vi "2D array to IMAQ.vi"(7 "Image Pixels (U8)":u8[][](array[numeric]), 8 "error in (no error)":errorcluster, 9 "Image Name":string="untitled", 10 "Image":T1, 11 "Thorcam in":refnum<class "Thorcam.lvclass">) -> (0 "error out":errorcluster, 2 "Image Name 2":string, 3 "Thorcam out":refnum<class "Thorcam.lvclass">, 4 "Image Out":T1)   [LabVIEW 2012, in "Thorcam.lvclass"]
uses:
  Thorcam.lvclass
  <vilib>/vision/Image Controls.llb/IMAQ Image.ctl
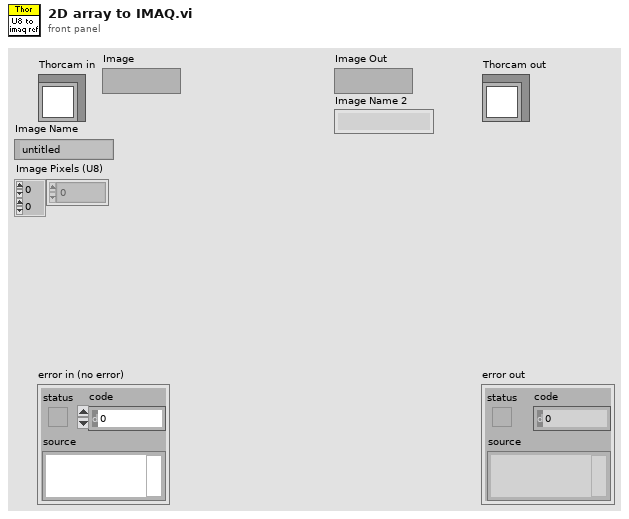
[diagram p1: front panel]
types:
  T1 = typedef "IMAQ Image.ctl" = refnum<image>
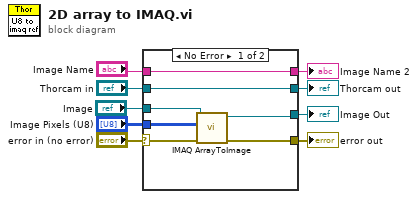
[diagram p0: block diagram]
diagram:
  n1 = case shown="No Error" "error in (no error)" {
    selector: "error in (no error)" -> [w11 w18]
    tunnel: [w16 w18] -> w8
    tunnel: [w13 w17] -> w6
    tunnel: "Thorcam in" -> [w13 w17]
    tunnel: "Image Name" -> [w12 _]
    tunnel: "Image Pixels (U8)" -> [w15 _]
    tunnel: [w14 _] -> w3
    tunnel: [w12 _] -> w2
    tunnel: "Image" -> [w10 _]
    frame No Error {
      n2 = call "IMAQ ArrayToImage"("error in (no error)"=w11, "Image Pixels (U8)"=w15, "Image"=w10) -> ("error out"=w16:errorcluster, "Image Out"=w14:T1)  [unwired: 7 in]
    }
    frame Error {
    }
  }
  "error out" <- w8
  "Thorcam out" <- w6
  "Image Out" <- w3
  "Image Name 2" <- w2
